vi "LJM logger exec SignedMSWLSW.vi"(8 "error in (no error)":errorcluster, 10 "LSB":dbl, 11 "MSB":dbl) -> (0 "error out":errorcluster, 3 "(MSB << 16 ) | LSB":i32)   [LabVIEW 2026]
doc: "Similar to the Formula Node function, but with variables that can be entered on the front panel."
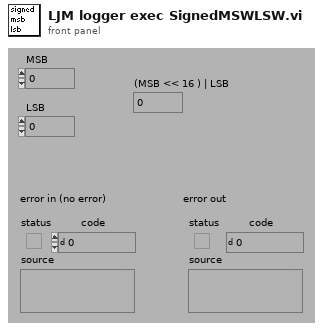
[diagram p1: front panel]
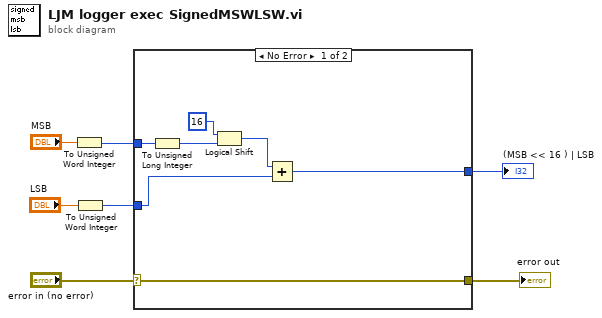
[diagram p0: block diagram]
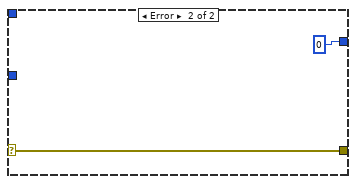
[diagram p2: hidden frame]
diagram:
  n1 = To Unsigned Word Integer(number="MSB") -> (unsigned 16bit integer=w2:u16)
  n2 = To Unsigned Word Integer(number="LSB") -> (unsigned 16bit integer=w4:u16)
  n3 = case shown="No Error" "error in (no error)" {
    selector: "error in (no error)" -> [w12 w16]
    tunnel: [w12 w16] -> w7
    tunnel: [w13 0] -> w5
    tunnel: w4 -> [w10 _]
    tunnel: w2 -> [w8 _]
    frame No Error {
      n4 = To Unsigned Long Integer(number=w8) -> (unsigned 32bit integer=w9:u32)
      n5 = Logical Shift(y=u32 16 ("x"), x=w9) -> (x << y=w14:u32)
      n6 = Add(x=w14, y=w10) -> (x+y=w13:u32)
    }
    frame Error {
    }
  }
  "error out" <- w7
  "(MSB << 16 ) | LSB" <- w5
